vi "ContAcq-IntClk.vi"() -> ()   [LabVIEW 2023]
uses:
  USB3202.dll
panel:
  in  "Enable":bool=TRUE caption="保存数据"
  out "Data":dbl[][](array[numeric])
  out "波形图":dbl[][](graph)
  in  "停止":bool
  in  "强制触发？":bool=TRUE
  in  "模拟通道触发":T1={"模拟触发使能"=FALSE, "触发方向"=0, "触发通道"=0, "触发电平V"=0.0, "触发灵敏度us"=1, "触发延迟点数"=0} {"触发通道" items=["AI0", "AI1", "AI2", "AI3", "AI4", "AI5", "AI6", "AI7"]; "触发方向" items=["下降沿", "上升沿", "变化"]}
  in  "外部数字触发":cluster{"数字触发使能":bool, "触发方向":u32} {"触发方向" items=["下降沿", "上升沿", "变化"]}
  in  "时钟参数配置":T2={"采样速率sps"=10000.0, "采样模式"=2, "每通道采样点数"=2048, "时钟源"=0, "时钟源输出？"=FALSE, "Reserve1"=0} {"时钟源" items=["内时钟", "外时钟"]; "采样模式" items=["单点采集", "有限点采集", "连续采集"]; "采样速率sps" min=1.0 max=250000.0 step=1.0 format="%#.7g"}
  in  "通道配置":T3(array[cluster])=[{"通道"=0, "增益"=0, "参考地"=0, "reserved0"=0, "reserved1"=0, "reserved2"=0}, {"通道"=1, "增益"=0, "参考地"=0, "reserved0"=0, "reserved1"=0, "reserved2"=0}, {"通道"=2, "增益"=0, "参考地"=0, "reserved0"=0, "reserved1"=0, "reserved2"=0}, {"通道"=3, "增益"=0, "参考地"=0, "reserved0"=0, "reserved1"=0, "reserved2"=0}, {"通道"=4, "增益"=0, "参考地"=0, "reserved0"=0, "reserved1"=0, "reserved2"=0}, {"通道"=5, "增益"=0, "参考地"=0, "reserved0"=0, "reserved1"=0, "reserved2"=0}, {"通道"=6, "增益"=0, "参考地"=0, "reserved0"=0, "reserved1"=0, "reserved2"=0}, {"通道"=7, "增益"=0, "参考地"=0, "reserved0"=0, "reserved1"=0, "reserved2"=0}] {"增益" items=["1倍增益", "2倍增益", "4倍增益", "8倍增益"]; "通道" items=["AI0", "AI1", "AI2", "AI3", "AI4", "AI5", "AI6", "AI7"]; "参考地" items=["参考单端", "非参考单端", "差分"]}
  in  "基础参数":T4 {"采样范围" items=["±10V", "±5V", "0-10V", "0-5V"]; "采样信号" items=["AI通道输入", "0V(AGND)", "2.5V"]; "采样通道数" items=["1", "2", "3", "4", "5", "6", "7", "8"]}
  # "注：line0代表使能的第一个通道，\n依次往下对应"
  # "注：每行代表使能的每个通道\n数据"
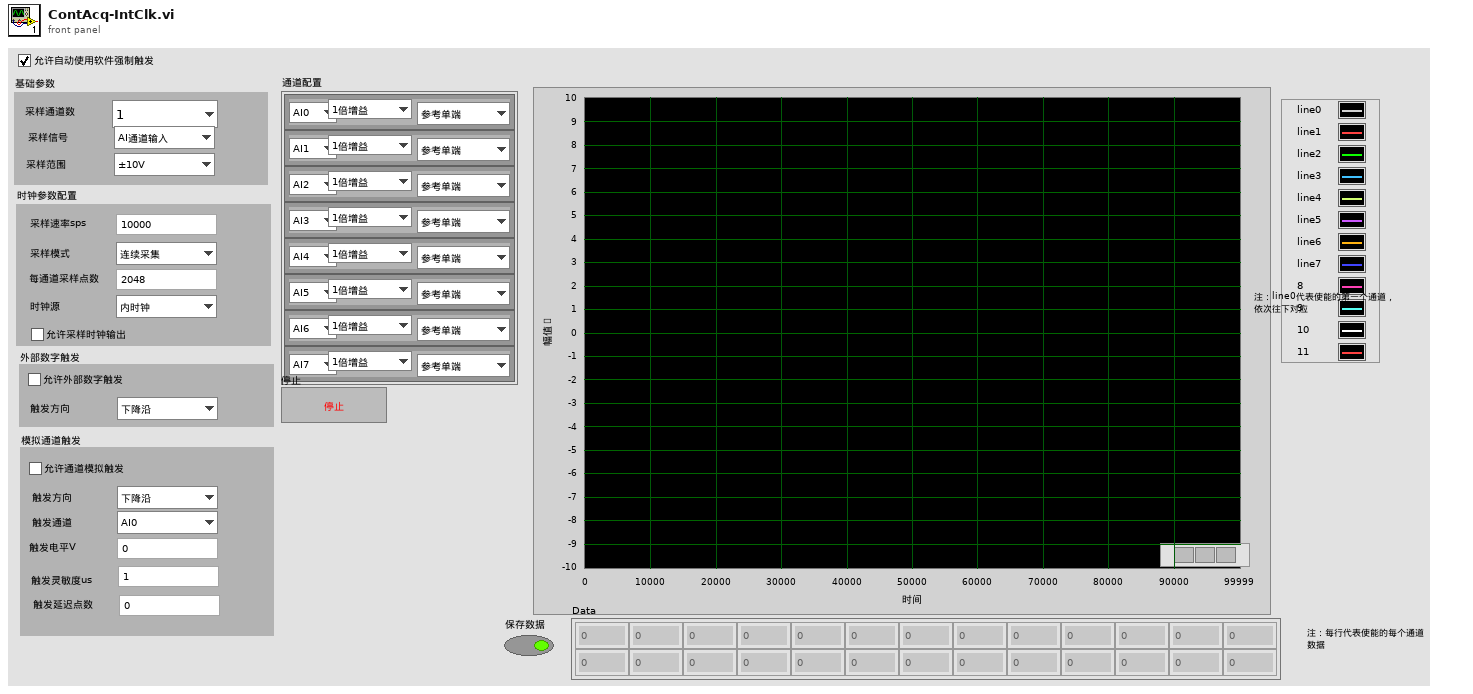
[diagram p1: front panel]
types:
  T1 = cluster{"模拟触发使能":bool, "触发方向":u32, "触发通道":u32, "触发电平V":sgl, "触发灵敏度us":u32, "触发延迟点数":u32}
  T2 = cluster{"采样速率sps":dbl, "采样模式":u32, "每通道采样点数":u32, "时钟源":u32, "时钟源输出？":bool, "Reserve1":u32}
  T3 = cluster{"通道":u32, "增益":u32, "参考地":u32, "reserved0":u32, "reserved1":u32, "reserved2":u32}[]
  T4 = cluster{"采样通道数":u32, "采样信号":u32, "采样范围":u32, "Reserve0":u32}
  T5 = cluster{"通道":u32, "增益":u32, "参考地":u32, "reserved0":u32, "reserved1":u32, "reserved2":u32}
  T6 = cluster{u32, "簇":cluster{"通道":u32, "增益":u32, "参考地":u32, "reserved0":u32, "reserved1":u32, "reserved2":u32}, "簇":cluster{"通道":u32, "增益":u32, "参考地":u32, "reserved0":u32, "reserved1":u32, "reserved2":u32}, "簇":cluster{"通道":u32, "增益":u32, "参考地":u32, "reserved0":u32, "reserved1":u32, "reserved2":u32}, "簇":cluster{"通道":u32, "增益":u32, "参考地":u32, "reserved0":u32, "reserved1":u32, "reserved2":u32}, "簇":cluster{"通道":u32, "增益":u32, "参考地":u32, "reserved0":u32, "reserved1":u32, "reserved2":u32}, "簇":cluster{"通道":u32, "增益":u32, "参考地":u32, "reserved0":u32, "reserved1":u32, "reserved2":u32}, "簇":cluster{"通道":u32, "增益":u32, "参考地":u32, "reserved0":u32, "reserved1":u32, "reserved2":u32}, "簇":cluster{"通道":u32, "增益":u32, "参考地":u32, "reserved0":u32, "reserved1":u32, "reserved2":u32}, "采样信号":u32, "采样范围":u32, "Reserve0":u32, "采样模式":u32, "每通道采样点数":u32, "采样速率sps":dbl, "时钟源":u32, u32, "Reserve1":u32, "Reserve1":u32, u32, "触发方向":u32, u32, "触发方向":u32, "触发通道":u32, "触发电平V":sgl, "触发灵敏度us":u32, "触发延迟点数":u32, u32, u32, u32, u32}
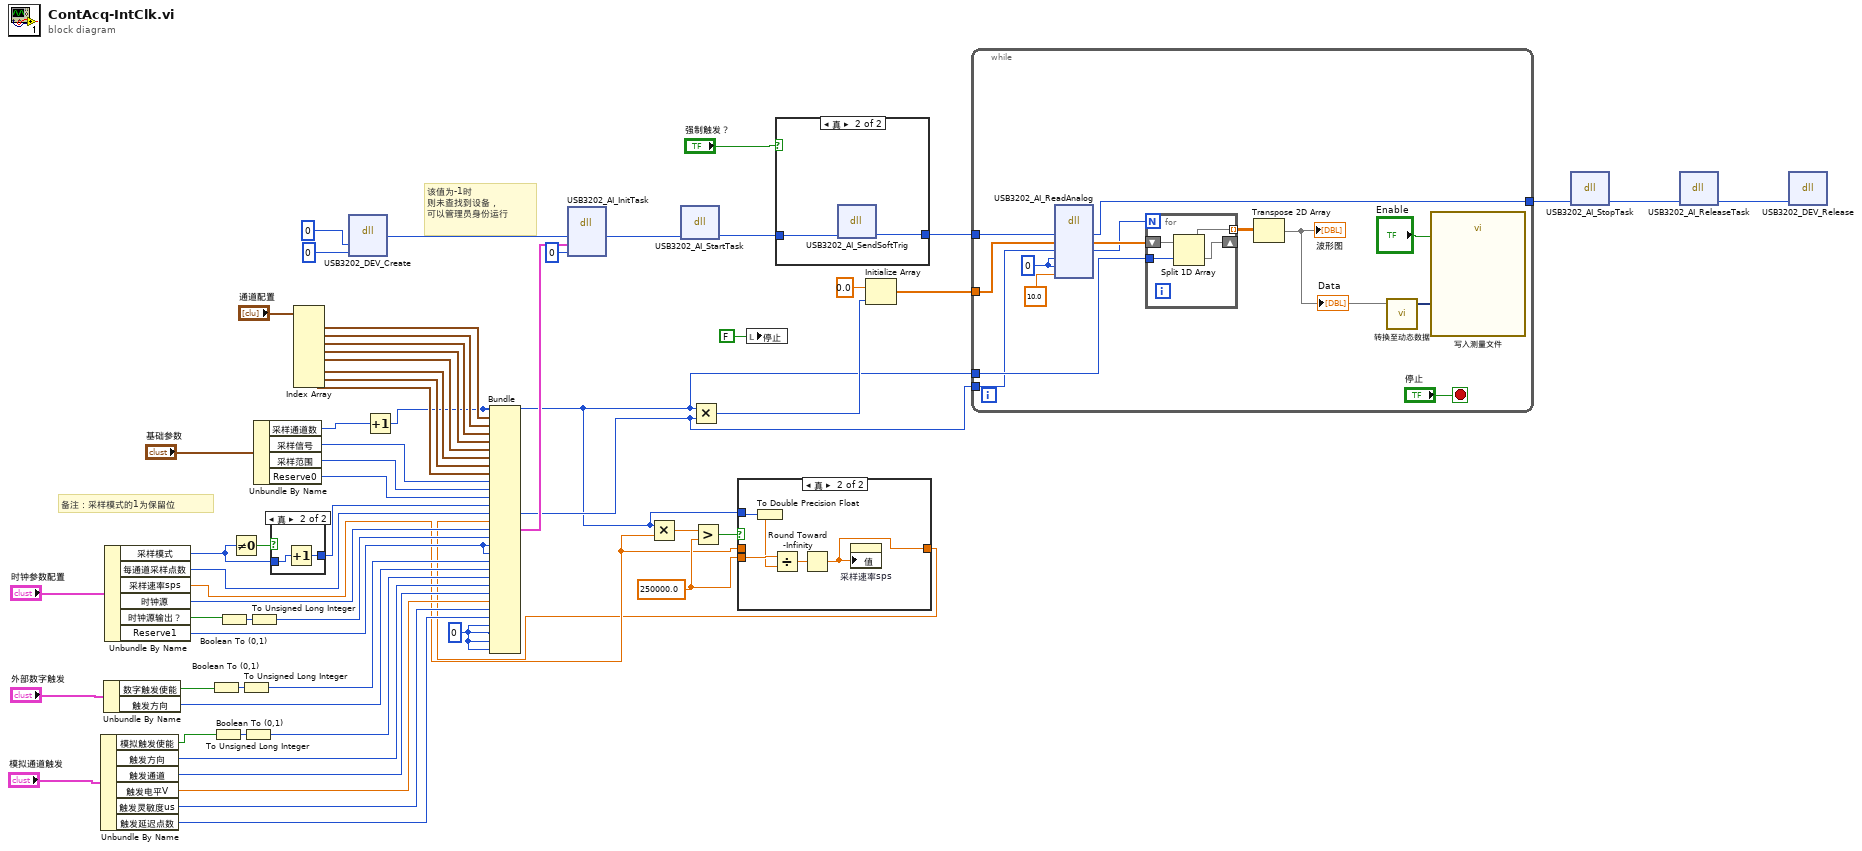
[diagram p0: block diagram]
diagram:
  w4 = 250000.0 ("y")
  w24 = u32 0
  # "该值为-1时\n则未查找到设备，\n可以管理员身份运行"
  # "备注：采样模式的1为保留位"
  n1 = Unbundle By Name("模拟通道触发") -> ("模拟触发使能"=w32:bool, "触发方向"=w30:u32, "触发通道"=w29:u32, "触发电平V"=w28:sgl, "触发灵敏度us"=w27:u32, "触发延迟点数"=w26:u32)
  n2 = Unbundle By Name("外部数字触发") -> ("数字触发使能"=w37:bool, "触发方向"=w35:u32)
  n3 = Unbundle By Name("时钟参数配置") -> ("采样模式"=w46:u32, "每通道采样点数"=w11:u32, "采样速率sps"=w2:dbl, "时钟源"=w44:u32, "时钟源输出？"=w42:bool, "Reserve1"=w40:u32)
  n4 = Boolean To (0,1)(Boolean=w37) -> (0, 1=w38:i16)
  n5 = Boolean To (0,1)(Boolean=w32) -> (0, 1=w33:i16)
  n6 = Boolean To (0,1)(Boolean=w42) -> (0, 1=w43:i16)
  n7 = Not Equal To 0?(x=w46) -> (x != 0?=w47:bool)
  n8 = To Unsigned Long Integer(number=w38) -> (unsigned 32bit integer=w36:u32)
  n9 = To Unsigned Long Integer(number=w33) -> (unsigned 32bit integer=w31:u32)
  n10 = To Unsigned Long Integer(number=w43) -> (unsigned 32bit integer=w41:u32)
  n11 = Unbundle By Name("基础参数") -> ("采样通道数"=w52:u32, "采样信号"=w51:u32, "采样范围"=w50:u32, "Reserve0"=w49:u32)
  n12 = case shown="真" w47 {
    tunnel: w46 -> [w62 w64]
    tunnel: [w62 w63] -> w45
    frame False {
    }
    frame True {
      n13 = Increment(x=w64) -> (x+1=w63:u32)
    }
  }
  n14 = Index Array(array="通道配置") -> (element #1=w59:T5, element #2=w58:T5, element #3=w57:T5, element #4=w56:T5, element #5=w55:T5, element #6=w54:T5, element #7=w53:T5, element #8=w25:T5)  [unwired: 8 in]
  n15 = dll-call lib="USB3202.dll" fn="USB3202_DEV_Create" label="DEV_Create"("nDeviceIdx"=u32 0, "bUsePhysIdx"=0) -> ("hDevice"=w20:i32)  [unwired: 5 in, 2 out]
  n16 = Increment(x=w52) -> (x+1=w3:u32)
  n17 = Multiply(x=w3, y=w2) -> (x*y=w6:dbl)
  n18 = Multiply(x=w3, y=w11) -> (x*y=w7:u32)
  n19 = Greater?(x=w6, y=w4) -> (0:w5:bool)
  n20 = case shown="真" w5 {
    tunnel: w4 -> [_ w70]
    tunnel: w3 -> [_ w69]
    tunnel: w2 -> [w65 _]
    tunnel: [w65 w66] -> w1
    frame False {
    }
    frame True {
      n21 = To Double Precision Float(number=w69) -> (double precision float=w68:dbl)
      n22 = Divide(x=w70, y=w68) -> (x/y=w67:dbl)
      n23 = Round Toward -Infinity(1:w67) -> (0:w66:dbl)
      n24 = property on="采样速率sps" class="DigNum (严格)"("值"=w66) -> ()  [unwired: 2 in, 2 out]
    }
  }
  n25 = Bundle(w3, "簇"=w59, "簇"=w58, "簇"=w57, "簇"=w56, "簇"=w55, "簇"=w54, "簇"=w53, "簇"=w25, "采样信号"=w51, "采样范围"=w50, "Reserve0"=w49, "采样模式"=w45, "每通道采样点数"=w11, "采样速率sps"=w1, "时钟源"=w44, w41, "Reserve1"=w40, "Reserve1"=w40, w36, "触发方向"=w35, w31, "触发方向"=w30, "触发通道"=w29, "触发电平V"=w28, "触发灵敏度us"=w27, "触发延迟点数"=w26, w24, w24, w24, w24) -> (w23:T6)  [unwired: 1 out]
  n26 = dll-call lib="USB3202.dll" fn="USB3202_AI_InitTask" label="InitTask"("hDevice"=w20, w23, "hEvent"=0) -> ("hDevice"=w18:i32)  [unwired: 4 in, 4 out]
  n27 = dll-call lib="USB3202.dll" fn="USB3202_AI_StartTask" label="AI_StartTask"("hDevice"=w18) -> ("hDevice"=w16:i32)  [unwired: 3 in, 3 out]
  n28 = local write "停止"(FALSE ("停止")) -> ()
  n29 = case shown="真" "强制触发？" {
    tunnel: w16 -> [w71 w73]
    tunnel: [w71 w72] -> w14
    frame False {
    }
    frame True {
      n30 = dll-call lib="USB3202.dll" fn="USB3202_AI_SendSoftTrig" label="SendSoftTrig"("hDevice"=w73) -> ("hDevice"=w72:i32)  [unwired: 3 in, 3 out]
    }
  }
  n31 = Initialize Array(0.0, w7) -> (w12:dbl[])
  n32 = while {
    tunnel: w14 -> [w84]
    tunnel: w12 -> [w82]
    tunnel: w3 -> [w81]
    tunnel: w11 -> [w78]
    tunnel: [w79] -> w9
    stop <- "停止" stop-if-true
    w85 = u32 0
    n33 = dll-call lib="USB3202.dll" fn="USB3202_AI_ReadAnalog" label="ReadBinary"("hDevice"=w84, "iBinaryArray"=w82, "nReadSampsPerChan"=w78, "pSampsPerChanRead"=w85, "pAvailSampsPerChan"=w85, "fTimeout"=10.0) -> ("hDevice"=w79:i32, "iBinaryArray"=w83:dbl[], "nReadSampsPerChan"=w77:u32)  [unwired: 4 in, 5 out]
    n34 = for {
      N: w77 -> [_]
      tunnel: w81 -> [w90]
      shift-right: [w89] -> _
      shift-left: w83 -> [w91]
      tunnel: [w88] -> w80 mode=indexing
      n35 = Split 1D Array(array=w91, index=w90) -> (first subarray=w88:dbl[], second subarray=w89:dbl[])
    }
    n36 = Transpose 2D Array(2D array=w80) -> (transposed array=w74:dbl[][])
    "波形图" <- w74
    "Data" <- w74
    n37 = call "转换至动态数据"("2D Array"=w74) -> ("Dynamic Data Type"=w76:dynamicdata)  [unwired: 3 in]
    n38 = call "写入测量文件"("Signals"=w76, "Enable"="Enable") -> ()  [unwired: 15 in, 3 out]
  }
  n39 = dll-call lib="USB3202.dll" fn="USB3202_AI_StopTask" label="AI_StopTask"("hDevice"=w9) -> ("hDevice"=w10:i32)  [unwired: 3 in, 3 out]
  n40 = dll-call lib="USB3202.dll" fn="USB3202_AI_ReleaseTask" label="AI_ReleaseTask"("hDevice"=w10) -> ("hDevice"=w8:i32)  [unwired: 3 in, 3 out]
  n41 = dll-call lib="USB3202.dll" fn="USB3202_DEV_Release"("hDevice"=w8) -> ()  [unwired: 4 in, 3 out]
